vi "D_FlipFlopWithReset 14.vi"(2 "________\nPresent":bool, 3 "______\nClear":bool, 4 "CLK":bool, 5 "D":bool) -> (0 "__\nQ":bool, 1 "Q":bool)   [LabVIEW 2018]
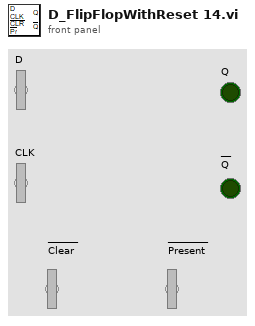
[diagram p1: front panel]
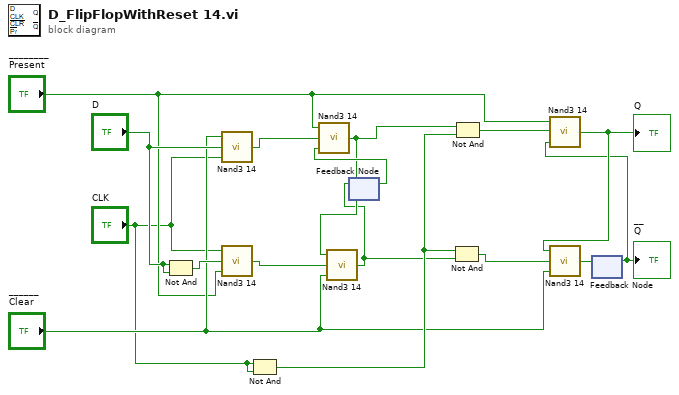
[diagram p0: block diagram]
diagram:
  n1 = Not And(1:"D", 2:"D") -> (0:w7:bool)
  n2 = call "Nand3 14.vi"("C"="CLK", "B"="D", "A"="______\nClear") -> ("Boolean"=w2:bool)
  n3 = call "Nand3 14.vi"("C"="________\nPresent", "B"=w7, "A"="CLK") -> ("Boolean"=w3:bool)
  n4 = Not And(1:"CLK", 2:"CLK") -> (0:w14:bool)
  n5 = feedback #1() -> (w16:bool)  [unwired: 1 in]
  n6 = call "Nand3 14.vi"("C"=w16, "B"=w2, "A"="________\nPresent") -> ("Boolean"=w15:bool)
  n7 = call "Nand3 14.vi"("C"="______\nClear", "B"=w3, "A"=w15) -> ("Boolean"=w13:bool)
  n8 = feedback-in #1(w13) -> ()
  n9 = Not And(1:w13, 2:w14) -> (0:w8:bool)
  n10 = Not And(1:w14, 2:w15) -> (0:w9:bool)
  n11 = feedback #2() -> (w10:bool)  [unwired: 1 in]
  "__\nQ" <- w10
  n12 = call "Nand3 14.vi"("C"=w10, "B"=w9, "A"="________\nPresent") -> ("Boolean"=w12:bool)
  "Q" <- w12
  n13 = call "Nand3 14.vi"("C"="______\nClear", "B"=w8, "A"=w12) -> ("Boolean"=w11:bool)
  n14 = feedback-in #2(w11) -> ()
